vi "HSV2RGB.vi"(9 "Value":dbl, 10 "Saturation":dbl=1.0, 11 "Hue [0-1)":dbl) -> (1 "Blue":u8, 2 "Green":u8, 3 "Red":u8)   [LabVIEW 2018]
doc: "Convert HSV to RGB Values. H is expressed as a value from 0-1, rather than 0-360. \n\n0= < H < 1"
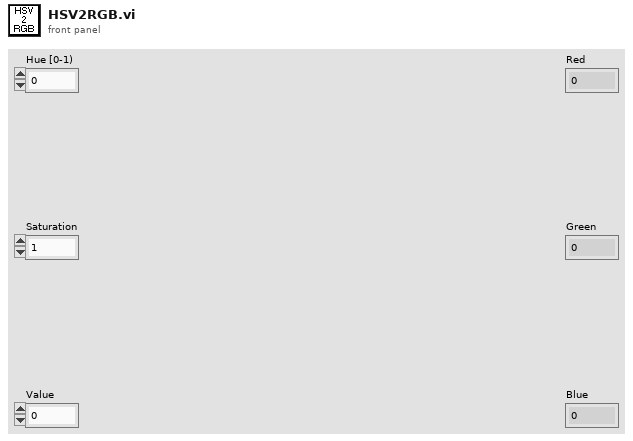
[diagram p1: front panel]
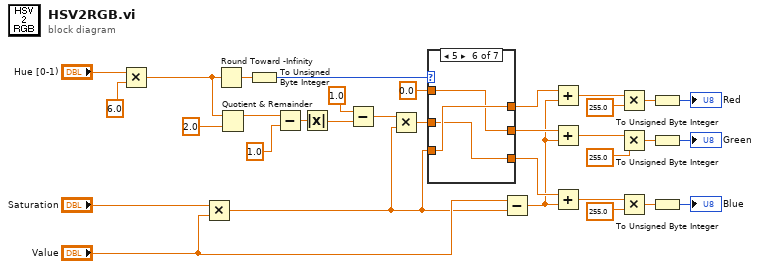
[diagram p0: block diagram]
diagram:
  n1 = Multiply(x="Hue [0-1)", y=6.0) -> (x*y=w8:dbl)
  n2 = Multiply(x="Saturation", y="Value") -> (x*y=w23:dbl)
  n3 = Round Toward -Infinity(1:w8) -> (0:w26:dbl)
  n4 = Quotient & Remainder(x=w8, y=2.0) -> (x-y*floor(x/y)=w6:dbl)  [unwired: 1 out]
  n5 = To Unsigned Byte Integer(number=w26) -> (unsigned 8bit integer=w9:u8)
  n6 = Subtract(x=w6, y=1.0) -> (x-y=w4:dbl)
  n7 = Absolute Value(x=w4) -> (abs(x)=w3:dbl)
  n8 = Subtract(x=1.0, y=w3) -> (x-y=w1:dbl)
  n9 = Multiply(x=w1, y=w23) -> (x*y=w25:dbl)
  n10 = case shown="5" w9 {
    tunnel: w23 -> [w36 w38 w41 w43 w46 w51 _]
    tunnel: w25 -> [w35 w39 w40 w44 w48 w49 _]
    tunnel: 0.0 -> [w34 w37 w42 w45 w47 w50 w52]
    tunnel: [w36 w39 w42 w45 w48 w51 w52] -> w20
    tunnel: [w35 w38 w41 w44 w47 w50 w52] -> w21
    tunnel: [w34 w37 w40 w43 w46 w49 w52] -> w22
    frame 0 {
    }
    frame 1 {
    }
    frame 2 {
    }
    frame 3 {
    }
    frame 4 {
    }
    frame 5 {
    }
    frame Default {
    }
  }
  n11 = Subtract(x="Value", y=w23) -> (x-y=w19:dbl)
  n12 = Add(x=w20, y=w19) -> (x+y=w10:dbl)
  n13 = Add(x=w21, y=w19) -> (x+y=w11:dbl)
  n14 = Add(x=w22, y=w19) -> (x+y=w12:dbl)
  n15 = Multiply(x=w10, y=255.0) -> (x*y=w17:dbl)
  n16 = Multiply(x=w11, y=255.0) -> (x*y=w16:dbl)
  n17 = Multiply(x=w12, y=255.0) -> (x*y=w14:dbl)
  n18 = To Unsigned Byte Integer(number=w17) -> (unsigned 8bit integer=→"Red":u8)
  n19 = To Unsigned Byte Integer(number=w16) -> (unsigned 8bit integer=→"Green":u8)
  n20 = To Unsigned Byte Integer(number=w14) -> (unsigned 8bit integer=→"Blue":u8)
